vi "LED Example LaunchPad.vi"() -> ()   [LabVIEW 2011]
panel:
  in  "Ring":u16(ring) items=["red"=0, "green"=6]
  in  "stop":bool
  in  "Dial Time Interval (ms)":u32(knob)=1004 scale=0.0..2000.0
  out "CurrentPath":path=path "C:/Documents and Settings/TGI0362/My Documents/xUserData/LabVIEW_8.x/cmDVT_Factory-BBU-R5"
  out "new picture":picture
  # "LED Toggle flashing \nwtih adjustable time delay"
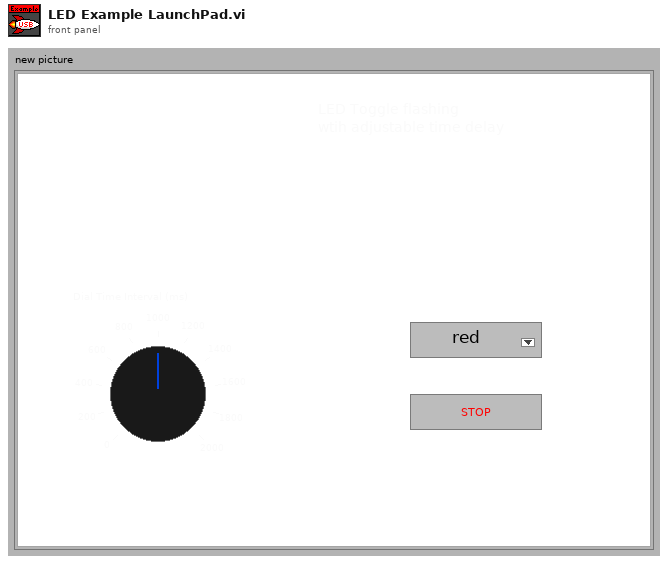
[diagram p1: front panel]
types:
  T1 = typedef "imagedata.ctl" = cluster{"image type":i32, "image depth":i32, "image":u8[], "mask":u8[], "colors":u32[], "Rectangle":cluster{"left":i16, "top":i16, "right":i16, "bottom":i16}}
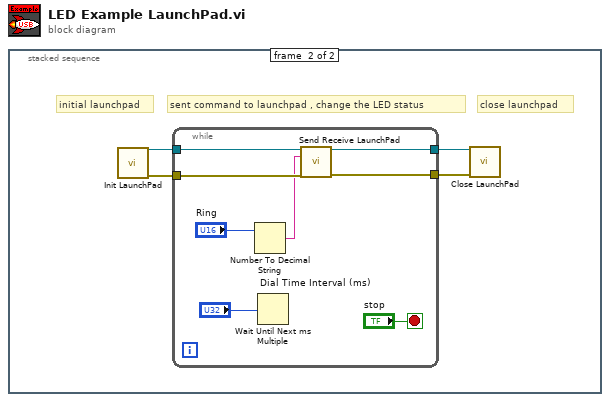
[diagram p0: block diagram]
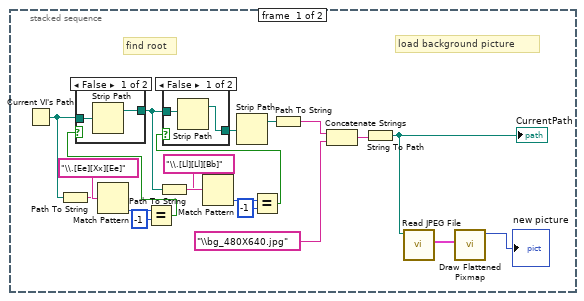
[diagram p2: hidden frame]
diagram:
  n1 = stacked-sequence {
    frame #0 {
      # "load background picture"
      # "find root"
      n2 = Current VI's Path() -> (path=w9:path)
      n3 = Path To String(path=w9) -> (string=w8:string)
      n4 = Match Pattern(string=w8, regular expression="\\.[Ee][Xx][Ee]") -> (offset past match=w6:i32)  [unwired: 1 in, 3 out]
      n5 = Equal?(x=w6, y=-1) -> (x = y?=w18:bool)
      n6 = case shown="False" w18 {
        tunnel: [w24 w26] -> w15
        tunnel: w9 -> [w25 w26]
        frame False {
          n7 = Strip Path(path=w25) -> (stripped path=w24:path)  [unwired: 1 out]
        }
        frame True {
        }
      }
      n8 = Path To String(path=w15) -> (string=w12:string)
      n9 = Match Pattern(string=w12, regular expression="\\.[Ll][Ll][Bb]") -> (offset past match=w14:i32)  [unwired: 1 in, 3 out]
      n10 = Equal?(x=w14, y=-1) -> (x = y?=w17:bool)
      n11 = case shown="False" w17 {
        tunnel: [w21 w23] -> w16
        tunnel: w15 -> [w22 w23]
        frame False {
          n12 = Strip Path(path=w22) -> (stripped path=w21:path)  [unwired: 1 out]
        }
        frame True {
        }
      }
      n13 = Strip Path(path=w16) -> (stripped path=w5:path)  [unwired: 1 out]
      n14 = Path To String(path=w5) -> (string=w2:string)
      n15 = Concatenate Strings(w2, "\\bg_480X640.jpg") -> (w3:string)
      n16 = String To Path(string=w3) -> (path=w1:path)
      "CurrentPath" <- w1
      n17 = call <vilib>:"Read JPEG File.vi"("path to JPEG file"=w1) -> ("image data"=w19:T1)  [unwired: 8 in, 2 out]
      n18 = call <vilib>:"Draw Flattened Pixmap.vi"("image data"=w19) -> ("new picture"=→"new picture":picture)  [unwired: 8 in]
    }
    frame #1 {
      # "close launchpad"
      # "sent command to launchpad , change the LED status"
      # "initial launchpad"
      n19 = call "Init LaunchPad.vi"() -> ("error out"=w27:errorcluster, "VISA resource name out"=w30:refnum<visa-resource-name>)  [unwired: 10 in]
      n20 = while {
        tunnel: w30 -> [w38]
        tunnel: [w37] -> w29
        tunnel: [w36] -> w28
        tunnel: w27 -> [w35]
        stop <- "stop" stop-if-true
        n21 = Number To Decimal String(number="Ring") -> (decimal integer string=w32:string)  [unwired: 1 in]
        n22 = Wait Until Next ms Multiple(millisecond multiple="Dial Time Interval (ms)") -> ()  [unwired: 1 out]
        n23 = call "Send Receive LaunchPad.vi"("VISA resource"=w38, "write buffer"=w32, "error in"=w35) -> ("VISA resource 2"=w37:refnum<visa-resource-name>, "error out"=w36:errorcluster)  [unwired: 10 in, 1 out]
      }
      n24 = call "Close LaunchPad.vi"("VISA resource name"=w29, "error in"=w28) -> ()  [unwired: 13 in, 1 out]
    }
  }
